vi "Get Object Refs from Node.vi"(8 "error in (no error)":errorcluster, 9 "refresh UI":T1, 11 "Data Value Reference in":T2) -> (0 "error out":errorcluster, 2 "refresh UI out":T1, 3 "references":T3)   [LabVIEW 2013, in "Scan Engine editor node.lvclass"]
doc: "Gets the reference to the engine and a generic Module Editor Node reference from the node we have. This will be used for operations in the UI."
uses:
  Scan Engine editor node.lvclass
  <vilib>/NI/DCAF/Tag Editor Core/Table API/Table Manager/object ref.ctl
  <vilib>/NI/DCAF/Tag Editor Core/Configuration Editor/Classes/Engine Parent/Engine Parent Editor Node.lvclass
  <vilib>/NI/DCAF/Tag Editor Core/Configuration Editor/Classes/Module editor node/module editor node.lvclass
  <vilib>/NI/Configuration Framework/Node/NodeRef.ctl
  <vilib>/NI/Configuration Framework/Node/NISE_CEF_Node.lvclass
  <vilib>/NI/Configuration Framework/Node/RefreshUIEvent.ctl
  <vilib>/NI/DCAF/Tag Editor Core/Table API/Table Manager/Table Manager.lvclass
  configuration/Scan Engine configuration.lvclass
  <vilib>/NI/Configuration Framework/serializable configuration/NISE_CEF_serializable configuration.lvclass
  <vilib>/NI/Module Execution Interface/Engine Configuration/engine configuration.lvclass
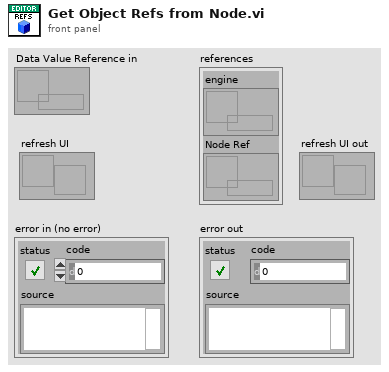
[diagram p1: front panel]
types:
  T1 = typedef "NISE_CEF_Node.lvclass/RefreshUIEvent.ctl" = refnum<user-event>
  T2 = typedef "NISE_CEF_Node.lvclass/NodeRef.ctl" = refnum<data-value>
  T3 = typedef "Table Manager.lvlib/Table Manager.lvclass/object ref.ctl" = cluster{"engine":refnum<data-value>, "Node Ref":refnum<data-value>}
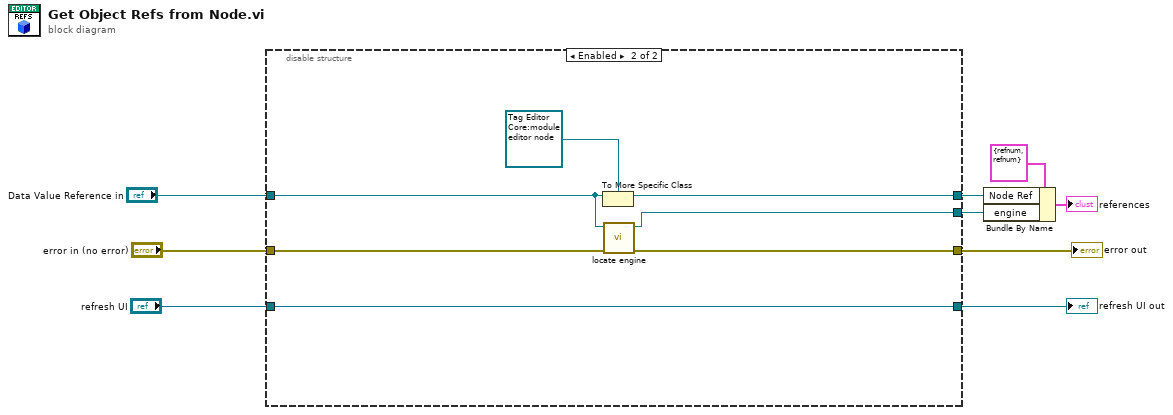
[diagram p0: block diagram]
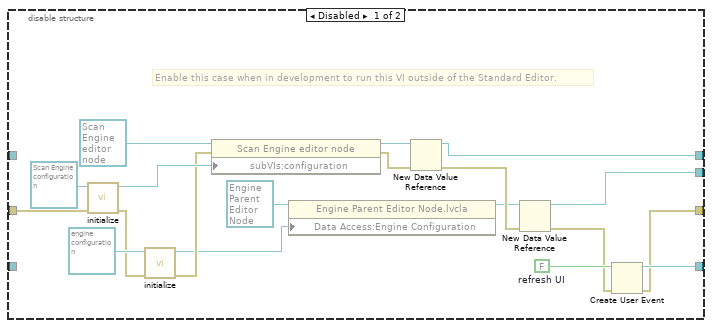
[diagram p2: hidden frame]
diagram:
  n1 = disable-structure shown="Enabled" {
    disable-tunnel: "Data Value Reference in" -> [_ w34]
    disable-tunnel: "error in (no error)" -> [w27 w33]
    disable-tunnel: [w10 w32] -> w5
    disable-tunnel: [w21 w31] -> w4
    disable-tunnel: [w17 w30] -> w3
    disable-tunnel: "refresh UI" -> [_ w29]
    disable-tunnel: [w18 w29] -> w1
    frame Disabled {
      w20 = FALSE  # refresh UI
      # "Enable this case when in development to run this VI outside of the Standard Editor."
      n2 = call <vilib>:"initialize.vi"("error in"=w27, "configuration in"=refnum<class "Scan Engine configuration.lvclass"> refnum ("tag bus configurable plugin module configuration")) -> ("error out"=w15:errorcluster, "configuration out"=w25:refnum<class "Scan Engine configuration.lvclass">)  [unwired: 7 in, 1 out]
      n3 = call <vilib>:"initialize.vi"("error in"=w15, "configuration in"=refnum<class "engine configuration.lvclass"> refnum ("engine configuration")) -> ("error out"=w14:errorcluster, "configuration out"=w12:refnum<class "engine configuration.lvclass">)  [unwired: 7 in, 1 out]
      n4 = property class="Scan Engine editor node"(reference=refnum<class "Scan Engine editor node.lvclass"> refnum ("Scan Engine editor node"), error in=w14, "subVIs:configuration"=w25) -> (reference out=w24:refnum<class "Scan Engine editor node.lvclass">, error out=w23:errorcluster)
      n5 = property class="Engine Parent Editor Node.lvcla"(reference=refnum<class "Engine Parent Editor Node.lvclass"> refnum ("PL Framework Configuration Tool.lvlib:Engine Parent Editor Node.lvclass"), "Data Access:Engine Configuration"=w12) -> (reference out=w11:refnum<class "Engine Parent Editor Node.lvclass">)  [unwired: 1 in, 1 out]
      n6 = New Data Value Reference(data value=w24, error in=w23) -> (data value reference=w10:refnum<data-value>, error out=w22:errorcluster)
      n7 = New Data Value Reference(data value=w11, error in=w22) -> (data value reference=w21:refnum<data-value>, error out=w19:errorcluster)
      n8 = Create User Event(user event datatype=w20, error in=w19) -> (user event=w18:refnum<user-event>, error out=w17:errorcluster)
    }
    frame Enabled {
      n9 = To More Specific Class(target class=refnum<data-value> refnum ("data value reference"), reference=w34) -> (specific class reference=w32:refnum<data-value>)  [unwired: 1 in, 1 out]
      n10 = call <vilib>:"locate engine.vi"("error in"=w33, "component"=w34) -> ("error out"=w30:errorcluster, "engine"=w31:refnum<data-value>)  [unwired: 8 in]
    }
  }
  "error out" <- w3
  "refresh UI out" <- w1
  n11 = Bundle By Name(cluster=T3 {"engine"=refnum, "Node Ref"=refnum} ("references"), "Node Ref"=w5, "engine"=w4) -> (→"references":T3)
